vi "Build Values Tree.vi"(7 "Tree":refnum<vi>, 9 "Types":T1[](array[typedef])) -> ()   [LabVIEW 2022 SP3, in "FlexBlocks Support.lvlib"]
uses:
  FlexBlocks Support.lvlib
  Type Descriptor.ctl
  Terminal Direction.ctl
  Value Mode.ctl
  Special Terminal.ctl
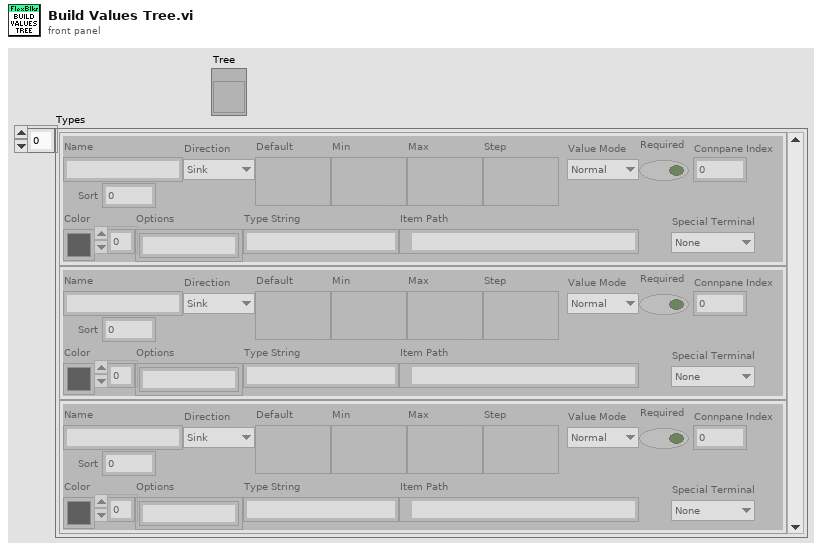
[diagram p1: front panel]
types:
  T1 = typedef "FlexBlocks Support.lvlib/Type Descriptor.ctl" = cluster{"Name":string, "Direction":T2, "Default":variant, "Min":variant, "Max":variant, "Step":variant, "Value Mode":T3, "Color":u32, "Options":string[], "Type String":string, "Item Path":path, "Required":bool, "Connpane Index":i32, "Special Terminal":T4, "Sort":i32}
  T2 = typedef "FlexBlocks Support.lvlib/Terminal Direction.ctl" = enum16{"Sink", "Source"}
  T3 = typedef "FlexBlocks Support.lvlib/Value Mode.ctl" = enum16{"Normal", "Range", "Select"}
  T4 = typedef "FlexBlocks Support.lvlib/Special Terminal.ctl" = enum16{"None", "Action", "Init", "Tag", "State in", "State out", "Error"}
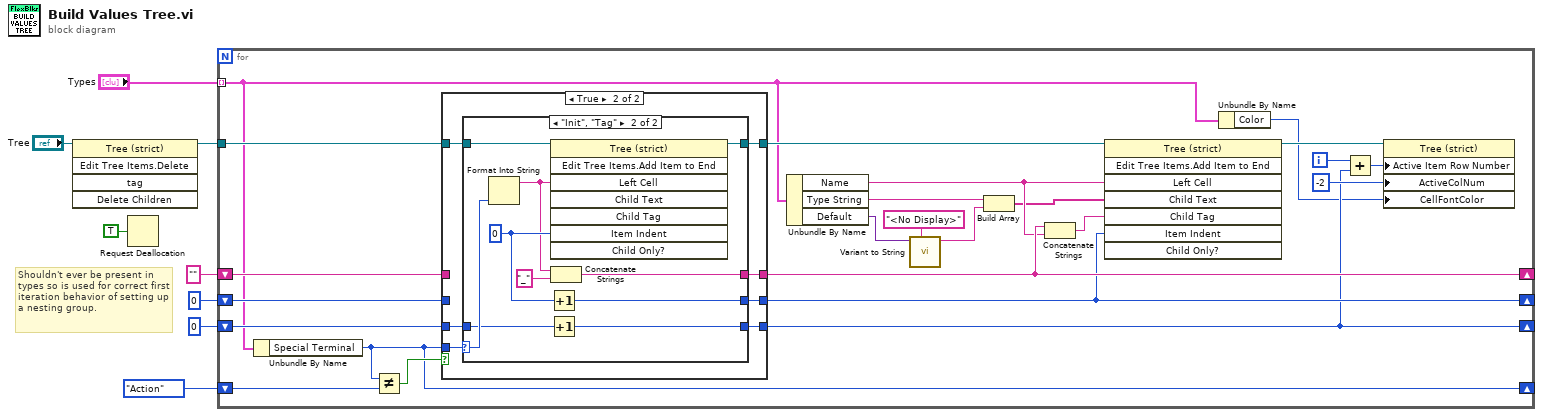
[diagram p0: block diagram]
diagram:
  # "Shouldn't ever be present in types so is used for correct first iteration behavior of setting up a nesting group."
  n1 = invoke class="Tree (strict)" method="Edit Tree Items.Delete"(reference="Tree") -> (reference out=w6:refnum<vi>)  [unwired: 4 in, 4 out]
  n2 = Request Deallocation(TRUE ("flag")) -> ()
  n3 = for {
    tunnel: w6 -> [w29]
    tunnel: "Types" -> [w15] mode=indexing
    shift-right: [w28] -> _
    shift-left: Special_Terminal."Action" ("Special Terminal") -> [w32]
    shift-right: [w11] -> _
    shift-left: 0 -> [w30]
    shift-right: [w20] -> _
    shift-left: "" -> [w27]
    shift-right: [w16] -> _
    shift-left: 0 -> [w26]
    i -> [w12]
    n4 = Unbundle By Name(w15) -> ("Special Terminal"=w28:T4)
    n5 = Not Equal?(x=w28, y=w32) -> (x != y?=w31:bool)
    n6 = case shown="True" w31 {
      tunnel: w28 -> [_ w43]
      tunnel: w30 -> [w33 w42]
      tunnel: [w33 w41] -> w11
      tunnel: [w34 w40] -> w16
      tunnel: [w35 w39] -> w20
      tunnel: w29 -> [w36 w38]
      tunnel: [w36 w37] -> w25
      tunnel: w27 -> [w35 _]
      tunnel: w26 -> [w34 _]
      frame False {
      }
      frame True {
        n7 = case shown="\"Init\", \"Tag\"" w43 {
          selector: w43 -> [_ w56]
          tunnel: w42 -> [w47 w53]
          tunnel: [w47 w52] -> w41
          tunnel: [0 w54] -> w40
          tunnel: ["" w49] -> w39
          tunnel: w38 -> [w44 w57]
          tunnel: [w44 w48] -> w37
          frame Default {
          }
          frame "Init", "Tag" {
            w55 = 0 ("New Item Indentation")
            n8 = Format Into String(w56) -> (resulting string=w50:string)  [unwired: 3 in, 1 out]
            n9 = Increment(x=w55) -> (x+1=w54:i32)
            n10 = Increment(x=w53) -> (x+1=w52:i32)
            n11 = invoke class="Tree (strict)" method="Edit Tree Items.Add Item to End"(reference=w57, "Left Cell"=w50, "Item Indent"=w55) -> (reference out=w48:refnum<vi>)  [unwired: 5 in, 7 out]
            n12 = Concatenate Strings(w50, "_" ("string")) -> (w49:string)
          }
        }
      }
    }
    n13 = Unbundle By Name(w15) -> ("Name"=w19:string, "Type String"=w22:string, "Default"=w24:variant)
    n14 = call "Variant to String.vi"("Unsupported (Empty)"="<No Display>", "Variant"=w24) -> ("String"=w21:string)  [unwired: 8 in, 1 out]
    n15 = Build Array(w22, w21) -> (w18:string[])
    n16 = Concatenate Strings(w20, w19) -> (w17:string)
    n17 = invoke class="Tree (strict)" method="Edit Tree Items.Add Item to End"(reference=w25, "Left Cell"=w19, "Child Text"=w18, "Child Tag"=w17, "Item Indent"=w16) -> (reference out=w14:refnum<vi>)  [unwired: 3 in, 7 out]
    n18 = Unbundle By Name(w15) -> ("Color"=w9:u32)
    n19 = Add(x=w12, y=w11) -> (x+y=w10:i32)
    n20 = property class="Tree (strict)"(reference=w14, "Active Item Row Number"=w10, "ActiveColNum"=-2 ("Active Cell:Active Column Number"), "CellFontColor"=w9) -> ()  [unwired: 1 in, 2 out]
  }
